vi "Get Panel Componnents Refs.vi"(8 "错误输入（无错误）":errorcluster, 11 "VI Ref In":refnum<vi>) -> (0 "错误输出":errorcluster, 1 "控件[]":refnum<vi>[](array[refnum]), 2 "窗格[]":refnum<vi>[](array[refnum]), 3 "VI Ref Out":refnum<vi>, 4 "修饰[]":refnum<vi>[](array[refnum]), 5 "所有对象[]":refnum<vi>[](array[refnum]), 6 "分隔栏[]":refnum<vi>[](array[refnum]))   [LabVIEW 2012, in "VIRef.lvlib"]
uses:
  VIRef.lvlib
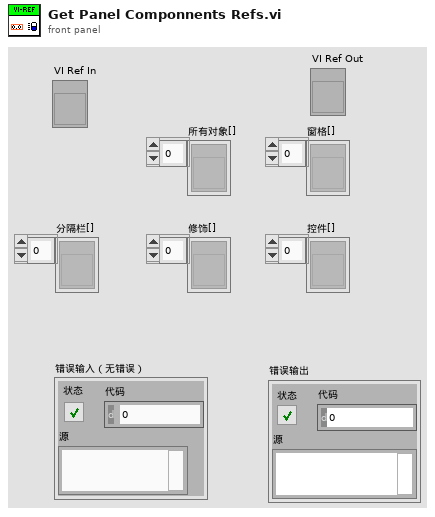
[diagram p1: front panel]
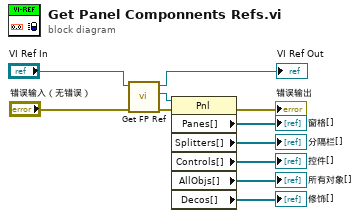
[diagram p0: block diagram]
diagram:
  n1 = call "Get FP Ref.vi"("错误输入（无错误）"="错误输入（无错误）", "VI Ref In"="VI Ref In") -> ("错误输出"=w9:errorcluster, "FP Ref"=w8:refnum<vi>, "VI Ref Out"=→"VI Ref Out":refnum<vi>)  [unwired: 7 in]
  n2 = property class="Pnl"(reference=w8, error in=w9) -> (error out=→"错误输出":errorcluster, "Panes[]"=→"窗格[]":refnum<vi>[], "Splitters[]"=→"分隔栏[]":refnum<vi>[], "Controls[]"=→"控件[]":refnum<vi>[], "AllObjs[]"=→"所有对象[]":refnum<vi>[], "Decos[]"=→"修饰[]":refnum<vi>[])  [unwired: 1 out]
